vi "Rotate_Block.vi"(10 "oldBlock":T1 {"orientaion" items=["up", "right", "down", "left"]; "type" items=["t", "rl", "ll", "rz", "lz", "square", "line"]}) -> (2 "newBlock":T1 {"orientaion" items=["up", "down", "left", "right"]; "type" items=["t", "rl", "ll", "rz", "lz", "square", "line"]})   [LabVIEW 2015]
uses:
  block.ctl
panel:
  in  "direction":dbl
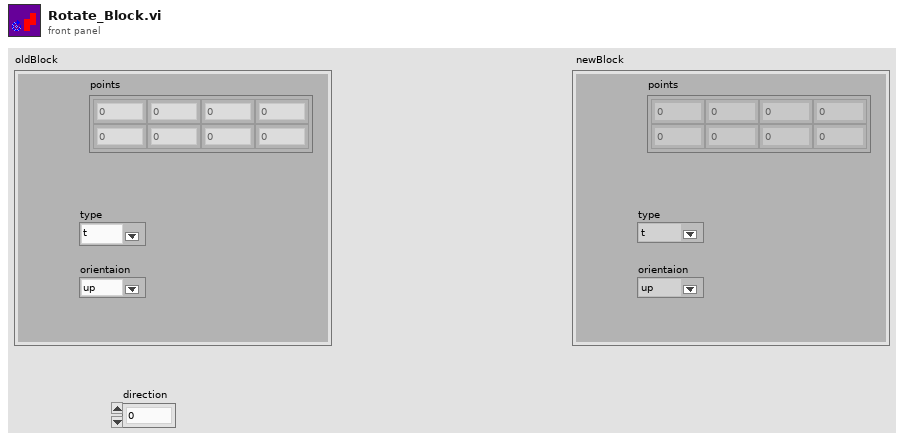
[diagram p1: front panel]
types:
  T1 = typedef "block.ctl" = cluster{"points":dbl[][], "type":u16, "orientaion":u16}
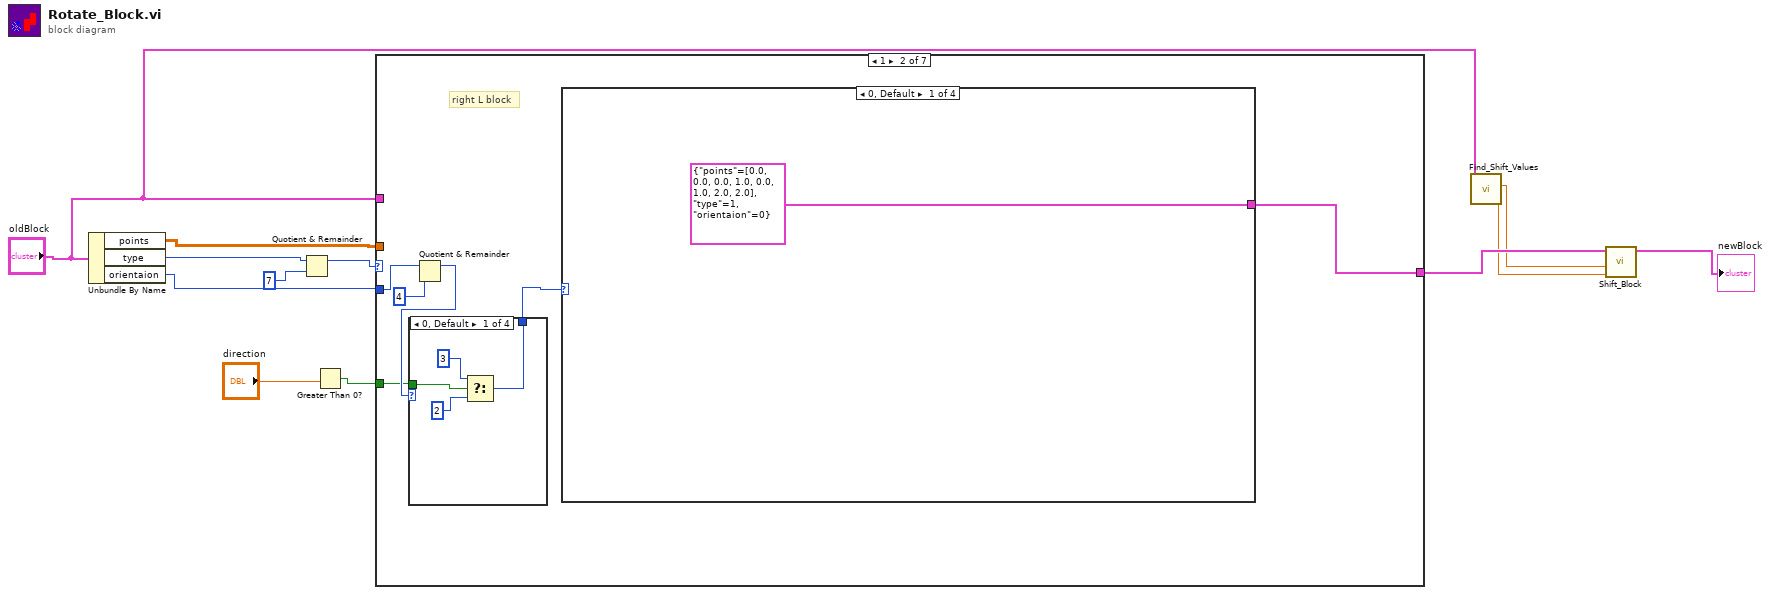
[diagram p0: block diagram]
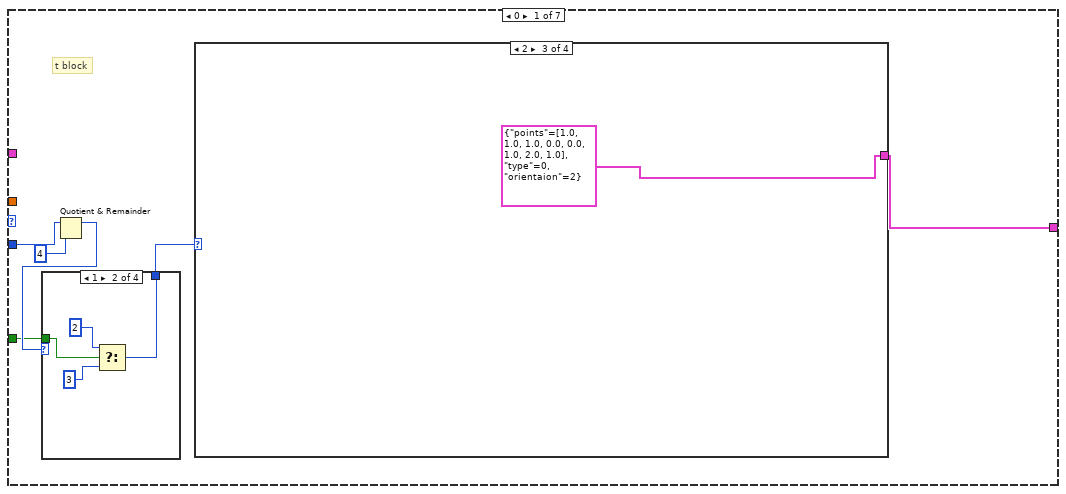
[diagram p2: hidden frame]
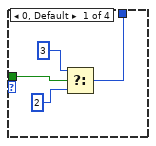
[diagram p3: hidden frame]
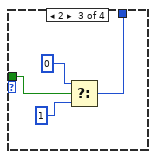
[diagram p4: hidden frame]
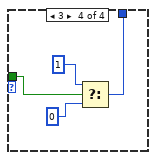
[diagram p5: hidden frame]
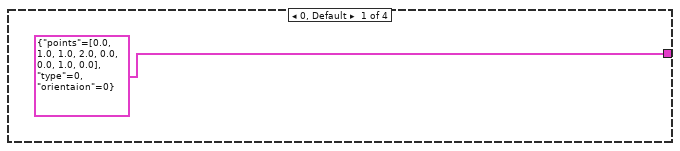
[diagram p6: hidden frame]
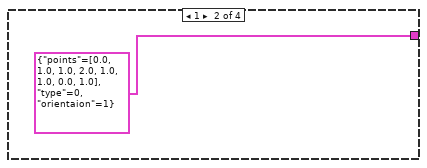
[diagram p7: hidden frame]
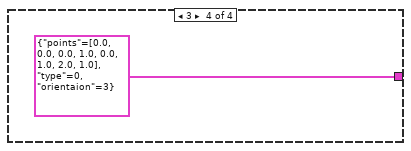
[diagram p8: hidden frame]
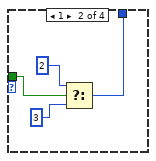
[diagram p9: hidden frame]
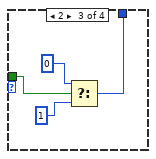
[diagram p10: hidden frame]
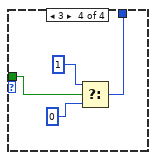
[diagram p11: hidden frame]
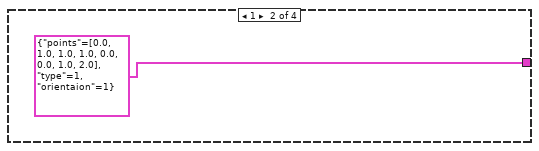
[diagram p12: hidden frame]
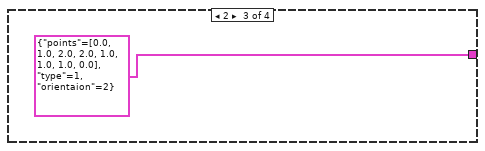
[diagram p13: hidden frame]
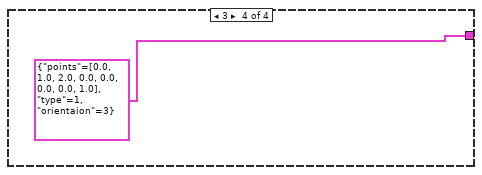
[diagram p14: hidden frame]
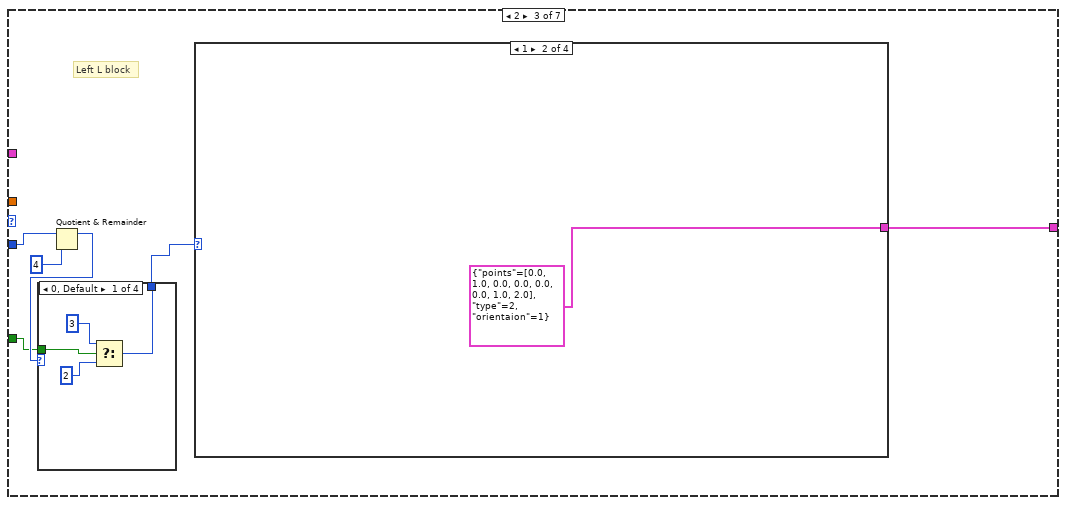
[diagram p15: hidden frame]
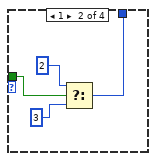
[diagram p16: hidden frame]
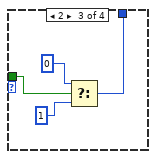
[diagram p17: hidden frame]
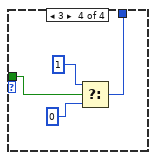
[diagram p18: hidden frame]
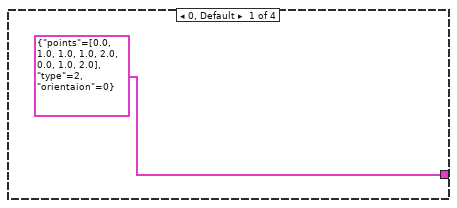
[diagram p19: hidden frame]
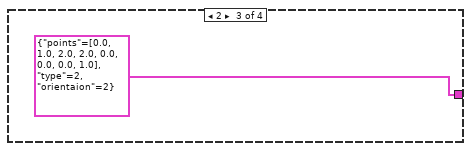
[diagram p20: hidden frame]
diagram:
  n1 = Unbundle By Name("oldBlock") -> ("points"=w12:dbl[][], "type"=w6:u16, "orientaion"=w11:u16)
  n2 = Quotient & Remainder(x=w6, y=7) -> (x-y*floor(x/y)=w8:i32)  [unwired: 1 out]
  n3 = Greater Than 0?(x="direction") -> (x > 0?=w9:bool)
  n4 = case shown="1" w8 {
    tunnel: w11 -> [w17 w40 w65 w93 w117 _ w147]
    tunnel: w12 -> [_ _ _ _ _ _ _]
    tunnel: "oldBlock" -> [_ _ _ _ _ _ _]
    tunnel: [w18 w44 w70 w96 w122 T1 {"points"=[[0.0, 0.0, 1.0, 1.0], [0.0, 1.0, 0.0, 1.0]], "type"=5, "orientaion"=0} ("Cluster") w149] -> w5
    tunnel: w9 -> [w14 w39 w66 w91 w119 _ w144]
    frame 0 {
      # "t block"
      n5 = Quotient & Remainder(x=w17, y=4) -> (x-y*floor(x/y)=w15:i32)  [unwired: 1 out]
      n6 = case shown="1" w15 {
        tunnel: w14 -> [w22 w24 w28 w31]
        tunnel: [w21 w23 w27 w32] -> w13
        frame 0, Default {
          n7 = Select(t=3, s=w22, f=2) -> (s? t:f=w21:i32)
        }
        frame 1 {
          n8 = Select(t=2, s=w24, f=3) -> (s? t:f=w23:i32)
        }
        frame 2 {
          n9 = Select(t=0, s=w28, f=1) -> (s? t:f=w27:i32)
        }
        frame 3 {
          n10 = Select(t=1, s=w31, f=0) -> (s? t:f=w32:i32)
        }
      }
      n11 = case shown="2" w13 {
        tunnel: [T1 {"points"=[[0.0, 1.0, 1.0, 2.0], [0.0, 0.0, 1.0, 0.0]], "type"=0, "orientaion"=0} ("Cluster") T1 {"points"=[[0.0, 1.0, 1.0, 2.0], [1.0, 1.0, 0.0, 1.0]], "type"=0, "orientaion"=1} ("Cluster") T1 {"points"=[[1.0, 1.0, 1.0, 0.0], [0.0, 1.0, 2.0, 1.0]], "type"=0, "orientaion"=2} ("Cluster") T1 {"points"=[[0.0, 0.0, 0.0, 1.0], [0.0, 1.0, 2.0, 1.0]], "type"=0, "orientaion"=3} ("Cluster")] -> w18
        frame 0, Default {
        }
        frame 1 {
        }
        frame 2 {
        }
        frame 3 {
        }
      }
    }
    frame 1 {
      # "right L block"
      n12 = Quotient & Remainder(x=w40, y=4) -> (x-y*floor(x/y)=w41:i32)  [unwired: 1 out]
      n13 = case shown="0, Default" w41 {
        tunnel: w39 -> [w48 w50 w54 w57]
        tunnel: [w47 w49 w53 w58] -> w42
        frame 0, Default {
          n14 = Select(t=3, s=w48, f=2) -> (s? t:f=w47:i32)
        }
        frame 1 {
          n15 = Select(t=2, s=w50, f=3) -> (s? t:f=w49:i32)
        }
        frame 2 {
          n16 = Select(t=0, s=w54, f=1) -> (s? t:f=w53:i32)
        }
        frame 3 {
          n17 = Select(t=1, s=w57, f=0) -> (s? t:f=w58:i32)
        }
      }
      n18 = case shown="0, Default" w42 {
        tunnel: [T1 {"points"=[[0.0, 0.0, 0.0, 1.0], [0.0, 1.0, 2.0, 2.0]], "type"=1, "orientaion"=0} ("Cluster") T1 {"points"=[[0.0, 1.0, 1.0, 1.0], [0.0, 0.0, 1.0, 2.0]], "type"=1, "orientaion"=1} ("Cluster") T1 {"points"=[[0.0, 1.0, 2.0, 2.0], [1.0, 1.0, 1.0, 0.0]], "type"=1, "orientaion"=2} ("Cluster") T1 {"points"=[[0.0, 1.0, 2.0, 0.0], [0.0, 0.0, 0.0, 1.0]], "type"=1, "orientaion"=3} ("Cluster")] -> w44
        frame 0, Default {
        }
        frame 1 {
        }
        frame 2 {
        }
        frame 3 {
        }
      }
    }
    frame 2 {
      # "Left L block"
      n19 = Quotient & Remainder(x=w65, y=4) -> (x-y*floor(x/y)=w67:i32)  [unwired: 1 out]
      n20 = case shown="0, Default" w67 {
        tunnel: w66 -> [w74 w76 w80 w83]
        tunnel: [w73 w75 w79 w84] -> w68
        frame 0, Default {
          n21 = Select(t=3, s=w74, f=2) -> (s? t:f=w73:i32)
        }
        frame 1 {
          n22 = Select(t=2, s=w76, f=3) -> (s? t:f=w75:i32)
        }
        frame 2 {
          n23 = Select(t=0, s=w80, f=1) -> (s? t:f=w79:i32)
        }
        frame 3 {
          n24 = Select(t=1, s=w83, f=0) -> (s? t:f=w84:i32)
        }
      }
      n25 = case shown="1" w68 {
        tunnel: [T1 {"points"=[[0.0, 1.0, 1.0, 1.0], [2.0, 0.0, 1.0, 2.0]], "type"=2, "orientaion"=0} ("Cluster") T1 {"points"=[[0.0, 1.0, 0.0, 0.0], [0.0, 0.0, 1.0, 2.0]], "type"=2, "orientaion"=1} ("Cluster") T1 {"points"=[[0.0, 1.0, 2.0, 2.0], [0.0, 0.0, 0.0, 1.0]], "type"=2, "orientaion"=2} ("Cluster") T1 {"points"=[[0.0, 0.0, 1.0, 2.0], [0.0, 1.0, 1.0, 1.0]], "type"=2, "orientaion"=3} ("Cluster")] -> w70
        frame 0, Default {
        }
        frame 1 {
        }
        frame 2 {
        }
        frame 3 {
        }
      }
    }
    frame 3 {
      # "right Z block"
      n26 = Quotient & Remainder(x=w93, y=4) -> (x-y*floor(x/y)=w92:i32)  [unwired: 1 out]
      n27 = case shown="0, Default" w92 {
        tunnel: w91 -> [w100 w102 w106 w109]
        tunnel: [w99 w101 w105 w110] -> w94
        frame 0, Default {
          n28 = Select(t=3, s=w100, f=2) -> (s? t:f=w99:i32)
        }
        frame 1 {
          n29 = Select(t=2, s=w102, f=3) -> (s? t:f=w101:i32)
        }
        frame 2 {
          n30 = Select(t=0, s=w106, f=1) -> (s? t:f=w105:i32)
        }
        frame 3 {
          n31 = Select(t=1, s=w109, f=0) -> (s? t:f=w110:i32)
        }
      }
      n32 = case shown="0, Default" w94 {
        tunnel: [T1 {"points"=[[0.0, 1.0, 1.0, 2.0], [1.0, 1.0, 0.0, 0.0]], "type"=3, "orientaion"=0} ("Cluster") T1 {"points"=[[0.0, 1.0, 1.0, 2.0], [1.0, 1.0, 0.0, 0.0]], "type"=3, "orientaion"=1} ("Cluster") T1 {"points"=[[0.0, 0.0, 1.0, 1.0], [0.0, 1.0, 1.0, 2.0]], "type"=3, "orientaion"=2} ("Cluster") T1 {"points"=[[0.0, 0.0, 1.0, 1.0], [0.0, 1.0, 1.0, 2.0]], "type"=3, "orientaion"=3} ("Cluster")] -> w96
        frame 0, Default {
        }
        frame 1 {
        }
        frame 2 {
        }
        frame 3 {
        }
      }
    }
    frame 4 {
      # "Left Z block"
      n33 = Quotient & Remainder(x=w117, y=4) -> (x-y*floor(x/y)=w118:i32)  [unwired: 1 out]
      n34 = case shown="0, Default" w118 {
        tunnel: w119 -> [w126 w128 w132 w135]
        tunnel: [w125 w127 w131 w136] -> w120
        frame 0, Default {
          n35 = Select(t=3, s=w126, f=2) -> (s? t:f=w125:i32)
        }
        frame 1 {
          n36 = Select(t=2, s=w128, f=3) -> (s? t:f=w127:i32)
        }
        frame 2 {
          n37 = Select(t=0, s=w132, f=1) -> (s? t:f=w131:i32)
        }
        frame 3 {
          n38 = Select(t=1, s=w135, f=0) -> (s? t:f=w136:i32)
        }
      }
      n39 = case shown="0, Default" w120 {
        tunnel: [T1 {"points"=[[0.0, 1.0, 1.0, 2.0], [0.0, 0.0, 1.0, 1.0]], "type"=4, "orientaion"=0} ("Cluster") T1 {"points"=[[0.0, 1.0, 1.0, 2.0], [0.0, 0.0, 1.0, 1.0]], "type"=4, "orientaion"=1} ("Cluster") T1 {"points"=[[0.0, 0.0, 1.0, 1.0], [1.0, 2.0, 1.0, 0.0]], "type"=4, "orientaion"=2} ("Cluster") T1 {"points"=[[0.0, 0.0, 1.0, 1.0], [1.0, 2.0, 1.0, 0.0]], "type"=4, "orientaion"=3} ("Cluster")] -> w122
        frame 0, Default {
        }
        frame 1 {
        }
        frame 2 {
        }
        frame 3 {
        }
      }
    }
    frame 5, Default {
      # "Square block"
    }
    frame 6 {
      # "L block"
      n40 = Quotient & Remainder(x=w147, y=4) -> (x-y*floor(x/y)=w145:i32)  [unwired: 1 out]
      n41 = case shown="0, Default" w145 {
        tunnel: w144 -> [w153 w155 w159 w162]
        tunnel: [w152 w154 w158 w163] -> w146
        frame 0, Default {
          n42 = Select(t=3, s=w153, f=2) -> (s? t:f=w152:i32)
        }
        frame 1 {
          n43 = Select(t=2, s=w155, f=3) -> (s? t:f=w154:i32)
        }
        frame 2 {
          n44 = Select(t=0, s=w159, f=1) -> (s? t:f=w158:i32)
        }
        frame 3 {
          n45 = Select(t=1, s=w162, f=0) -> (s? t:f=w163:i32)
        }
      }
      n46 = case shown="3" w146 {
        tunnel: [T1 {"points"=[[0.0, 0.0, 0.0, 0.0], [0.0, 1.0, 2.0, 3.0]], "type"=6, "orientaion"=0} ("Cluster") T1 {"points"=[[0.0, 0.0, 0.0, 0.0], [0.0, 1.0, 2.0, 3.0]], "type"=6, "orientaion"=1} ("Cluster") T1 {"points"=[[0.0, 1.0, 2.0, 3.0], [0.0, 0.0, 0.0, 0.0]], "type"=6, "orientaion"=2} ("Cluster") T1 {"points"=[[0.0, 1.0, 2.0, 3.0], [0.0, 0.0, 0.0, 0.0]], "type"=6, "orientaion"=3} ("Cluster")] -> w149
        frame 0, Default {
        }
        frame 1 {
        }
        frame 2 {
        }
        frame 3 {
        }
      }
    }
  }
  n47 = call "Find_Shift_Values.vi"("Block"="oldBlock") -> ("y-value"=w3:dbl, "x-value"=w4:dbl)  [unwired: 9 in]
  n48 = call "Shift_Block.vi"("y"=w3, "x"=w4, "old"=w5) -> ("new"=→"newBlock":T1)  [unwired: 8 in]
